vi "ReadI64.vi"(11 "Address":u32) -> (3 "Data":i64)   [LabVIEW 2016]
uses:
  <vilib>/rvi/Memory/Memory_Emulation/nirvimemoryFastEmulation.vi
  <vilib>/rvi/Memory/Memory_Emulation/nirvimemoryEmulation.vi
  <vilib>/rvi/Emulation/niFpgaEmulationIsFPGAContextNoSignature.vi
  <vilib>/rvi/DataTransferAndStorage/Container/Common/niFpgaContainerGetUniqueNameForEmu.vi
  <vilib>/rvi/Emulation/niFpgaProcessEmulError.vi
  <vilib>/rvi/Emulation/niFpgaSctlEmulationGetInTimedLoop.vi
  <vilib>/rvi/errors/nirviReportUnexpectedCaseInternalError (U32).vi
  <vilib>/rvi/DataTransferAndStorage/Container/Common/niFpgaContainerExecOnDevCompGetState.vi
  <vilib>/rvi/Memory/Memory_Emulation/niFpgaMemoryEmulationCacheClearOnFirstRun.vi
  <vilib>/rvi/Memory/Memory_Emulation/nirvimemoryEmulationManagerCache_MakeExclusive.vi
  <vilib>/rvi/Memory/Memory_Emulation/niFpgaMemoryEmulationValidateCache.vi
  <vilib>/rvi/Memory/Memory_Emulation/nirvimemoryEmulationManagerCache_InsertValue.vi
  <vilib>/Utility/error.llb/Clear Errors.vi
  <vilib>/rvi/Memory/Memory_Emulation/nirvimemoryEmulationManagerCache_ReleaseExclusive.vi
  <vilib>/rvi/Memory/Memory_Emulation/nirvimemoryEmulationManagerCache_GetValue.vi
  <vilib>/rvi/Memory/Memory_Emulation/nirvimemoryEmulationManagerCache_SetValue.vi
  <vilib>/rvi/Emulation/niFpgaSctlEmulationResourceMgr.vi
  <vilib>/rvi/DataTransferAndStorage/Container/XNode/niFpgaContainer.xnode
  <vilib>/rvi/Memory/Memory_Emulation/niFpgaMemoryEmulationRefIn.vi
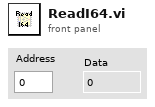
[diagram p1: front panel]
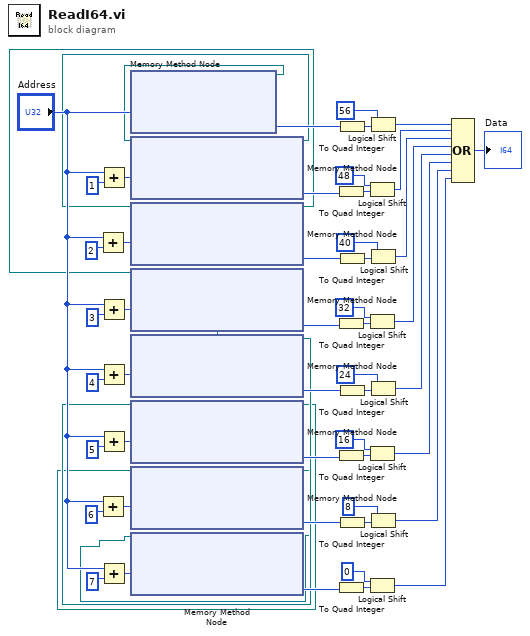
[diagram p0: block diagram]
diagram:
  n1 = Add(x="Address", y=u32 2) -> (x+y=w35:u32)
  n2 = Add(x="Address", y=u32 6) -> (x+y=w32:u32)
  n3 = Add(x="Address", y=u32 1) -> (x+y=w45:u32)
  n4 = Add(x="Address", y=u32 3) -> (x+y=w44:u32)
  n5 = Add(x="Address", y=u32 4) -> (x+y=w13:u32)
  n6 = Add(x="Address", y=u32 5) -> (x+y=w22:u32)
  n7 = Add(x="Address", y=u32 7) -> (x+y=w23:u32)
  n8 = xnode ("Memory Method Node")("Address"="Address") -> ("Data"=w55:u8, "Memory Out"=w7:refnum<k21>)  [unwired: 1 in]
  n9 = xnode ("Memory Method Node")("Address"=w45, "Memory In"=w7) -> ("Data"=w50:u8, "Memory Out"=w6:refnum<k21>)
  n10 = xnode ("Memory Method Node")("Address"=w35, "Memory In"=w6) -> ("Data"=w37:u8, "Memory Out"=w5:refnum<k21>)
  n11 = xnode ("Memory Method Node")("Address"=w44, "Memory In"=w5) -> ("Data"=w41:u8, "Memory Out"=w4:refnum<k21>)
  n12 = xnode ("Memory Method Node")("Address"=w13, "Memory In"=w4) -> ("Data"=w15:u8, "Memory Out"=w3:refnum<k21>)
  n13 = xnode ("Memory Method Node")("Address"=w22, "Memory In"=w3) -> ("Data"=w19:u8, "Memory Out"=w2:refnum<k21>)
  n14 = xnode ("Memory Method Node")("Address"=w32, "Memory In"=w2) -> ("Data"=w30:u8, "Memory Out"=w1:refnum<k21>)
  n15 = xnode ("Memory Method Node")("Address"=w23, "Memory In"=w1) -> ("Data"=w26:u8)  [unwired: 1 out]
  n16 = To Quad Integer(1:w50) -> (0:w51:i64)
  n17 = To Quad Integer(1:w41) -> (0:w40:i64)
  n18 = To Quad Integer(1:w19) -> (0:w18:i64)
  n19 = To Quad Integer(1:w26) -> (0:w27:i64)
  n20 = To Quad Integer(1:w55) -> (0:w54:i64)
  n21 = To Quad Integer(1:w37) -> (0:w38:i64)
  n22 = To Quad Integer(1:w15) -> (0:w16:i64)
  n23 = To Quad Integer(1:w30) -> (0:w29:i64)
  n24 = Logical Shift(y=i16 48, x=w51) -> (x << y=w48:i64)
  n25 = Logical Shift(y=i16 32, x=w40) -> (x << y=w33:i64)
  n26 = Logical Shift(y=i16 16, x=w18) -> (x << y=w10:i64)
  n27 = Logical Shift(y=i16 0, x=w27) -> (x << y=w8:i64)
  n28 = Logical Shift(y=i16 56, x=w54) -> (x << y=w52:i64)
  n29 = Logical Shift(y=i16 40, x=w38) -> (x << y=w34:i64)
  n30 = Logical Shift(y=i16 24, x=w16) -> (x << y=w11:i64)
  n31 = Logical Shift(y=i16 8, x=w29) -> (x << y=w9:i64)
  n32 = Compound Arithmetic op=OR(w52, w48, w34, w33, w11, w10, w9, w8) -> (→"Data":i64)
